vi "test.vi"() -> ()   [LabVIEW 2015]
uses:
  <vilib>/rvi/Emulation/niFpgaGetClockAttributes.vi
  <vilib>/rvi/Emulation/niFpgaSctlEmulationGetInTimedLoop.vi
  <vilib>/rvi/Emulation/niFpgaEmulationReportErrorSimple.vi
  <vilib>/rvi/eio/common/nirviEmuTemplateMethod_errors.vi
  <vilib>/rvi/Emulation/niFpgaCriticalErrorInLSC.vi
  <vilib>/eio/EIONode/EIONode.xnode
panel:
  in  "Boolean":bool
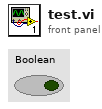
[diagram p1: front panel]
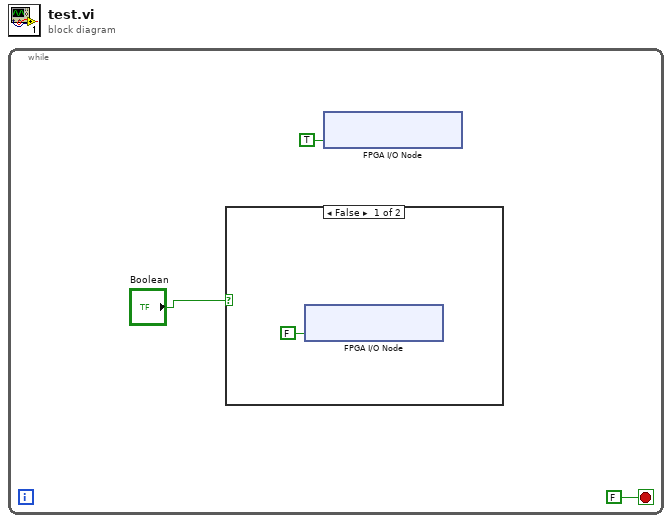
[diagram p0: block diagram]
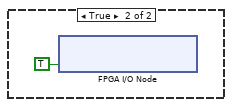
[diagram p2: hidden frame]
diagram:
  n1 = while {
    stop <- FALSE stop-if-true
    n2 = case shown="False" "Boolean" {
      frame False {
        n3 = xnode "FPGA I/O Node"("ConnectorC/DIO3"=FALSE ("ConnectorC/DIO4")) -> ()  [unwired: 1 in, 1 out]
      }
      frame True {
        n4 = xnode "FPGA I/O Node"("ConnectorC/DIO3"=TRUE ("ConnectorC/DIO4")) -> ()  [unwired: 1 in, 1 out]
      }
    }
    n5 = xnode "FPGA I/O Node"("ConnectorC/DIO4"=TRUE) -> ()  [unwired: 1 in, 1 out]
  }
